vi "Save VI Image.vi"(8 "error in (no error)":errorcluster, 10 "Image Path":path, 11 "VI in":refnum<vi>) -> (0 "error out":errorcluster, 3 "VI out":refnum<vi>)   [LabVIEW 2020]
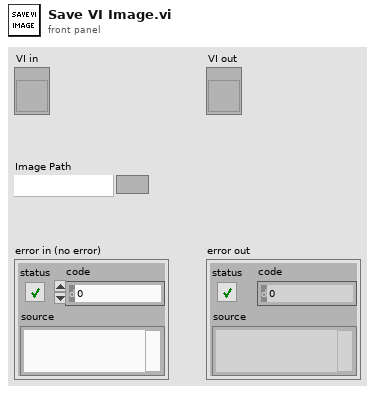
[diagram p1: front panel]
types:
  T1 = typedef "imagedata.ctl" = cluster{"image type":i32, "image depth":i32, "image":u8[], "mask":u8[], "colors":u32[], "Rectangle":cluster{"left":i16, "top":i16, "right":i16, "bottom":i16}}
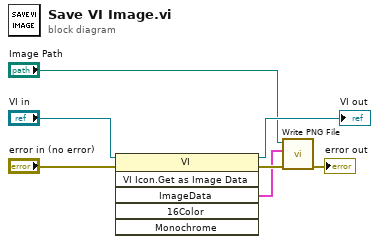
[diagram p0: block diagram]
diagram:
  n1 = invoke class="VI" method="VI Icon.Get as Image Data"(reference="VI in", error in="error in (no error)") -> (reference out=→"VI out":refnum<vi>, error out=w6:errorcluster, "ImageData"=w1:T1)  [unwired: 4 in, 3 out]
  n2 = call <vilib>:"Write PNG File.vi"("error in (no error)"=w6, "image data"=w1, "path to PNG file"="Image Path") -> ("error out"=→"error out":errorcluster)  [unwired: 7 in, 1 out]
